vi "h.ACQ.GetSpectrum.vi"(6 "power scales and offsets":i32[][](array[numeric]), 8 "error in":errorcluster, 9 "Single Channel":u8=1 min=1 max=16 step=1, 10 "All Channels":bool, 11 "Connection ID In":refnum<k5>) -> (0 "error out":errorcluster, 2 "Spectral Data":T1={"Spectrum"=[{"Spectrum, db"=array[32000 elements]}, {"Spectrum, db"=[]}, {"Spectrum, db"=[]}, {"Spectrum, db"=[]}, {"Spectrum, db"=[]}, {"Spectrum, db"=[]}, {"Spectrum, db"=[]}, {"Spectrum, db"=[]}, {"Spectrum, db"=[]}, {"Spectrum, db"=[]}, {"Spectrum, db"=[]}, {"Spectrum, db"=[]}, {"Spectrum, db"=[]}, {"Spectrum, db"=[]}, {"Spectrum, db"=[]}, {"Spectrum, db"=[]}], "Start Wvl"=1460.0, "Wvl Inc"=0.005, "SN"=96718, "Time Stamp (ns)"=1308286670531232440} {"Spectrum"."Spectrum, db" format="%_8g"}, 3 "Connection ID Out":refnum<k5>)   [LabVIEW 2019, in "h.Library.lvlib"]
doc: "This VI retrieves spectral plots from a Hyperion instrument.\n\n<b>Connection ID</b> - is a network connection refnum that uniquely identifies the TCP connection\n<b>Timeout</b> - specifies the maximum amount of time, in milliseconds, for the function to complete\n<b>Channel</b> - specifies the spectrum channel number (1-16)\n<b>error in</b> - describes error conditions that occur before this node runs. This input provides standard error functionality\n<b>Connection ID out</b> - returns the same value as connection ID\n<b>Spectral Data</b> - cluster containing requested spectrum along with supporting data\n<b>error out</b> - contains error information. This output provides standard error out functionality."
uses:
  h.Library.lvlib
  CTL/h.ACQ.SpectralData.ctl
  CTL/h.ACQ.Spectrum.ctl
panel:
  # "Hyperion #GetSpectrum"
  # "OR"
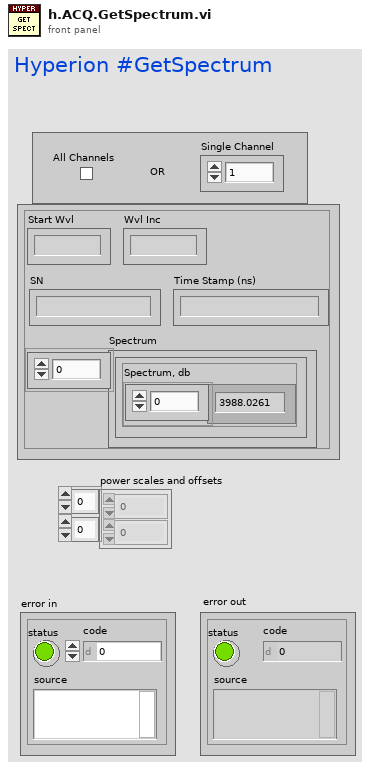
[diagram p1: front panel]
types:
  T1 = typedef "h.Library.lvlib/h.ACQ.SpectralData.ctl" = cluster{"Spectrum":T2[], "Start Wvl":dbl, "Wvl Inc":dbl, "SN":u64, "Time Stamp (ns)":u64}
  T2 = typedef "h.Library.lvlib/h.ACQ.Spectrum.ctl" = cluster{"Spectrum, db":dbl[]}
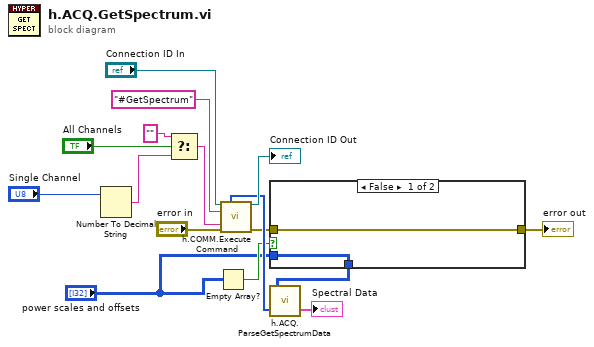
[diagram p0: block diagram]
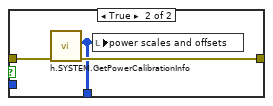
[diagram p2: hidden frame]
diagram:
  n1 = Number To Decimal String(number="Single Channel") -> (decimal integer string=w5:string)  [unwired: 1 in]
  n2 = Select(t="", s="All Channels", f=w5) -> (s? t:f=w3:string)
  n3 = Empty Array?(array="power scales and offsets") -> (empty?=w9:bool)
  n4 = call "h.COMM.Execute Command.vi"("Connection ID"="Connection ID In", "Command"="#GetSpectrum", "Argument"=w3, "error in"="error in") -> ("Content"=w11:u8[], "Connection ID out"=→"Connection ID Out":refnum<k5>, "error out"=w8:errorcluster)  [unwired: 4 in, 5 out]
  n5 = case shown="False" w9 {
    tunnel: w8 -> [w18 w21]
    tunnel: [w18 w20] -> w7
    tunnel: [w17 w19] -> w2
    tunnel: "power scales and offsets" -> [w17 _]
    frame False {
    }
    frame True {
      n6 = call "h.SYSTEM.GetPowerCalibrationInfo.vi"("error in"=w21) -> ("error out"=w20:errorcluster, "power scales and offsets"=w19:i32[][])  [unwired: 8 in, 1 out]
      n7 = local write "power scales and offsets"(w19) -> ()
    }
  }
  "error out" <- w7
  n8 = call "h.ACQ.ParseGetSpectrumData.vi"("Data from #GetSpectrum"=w11, "power scales and offsets"=w2) -> ("Spectral Data"=→"Spectral Data":T1)  [unwired: 1 in]
